vi "Rename Selected Waveform.vi"(8 "error in (no error)":errorcluster, 9 "New Waveform Name":string, 10 "Waveform Listbox Ref":refnum<vi>, 11 "Data In":T1 {"Toggle Channels"."Initial State" items=["High"=101, "Low"=102]; "Sample Rate" format="%.2p"}) -> (0 "error out":errorcluster, 3 "Data Out":T1 {"Toggle Channels"."Initial State" items=["High"=101, "Low"=102]; "Sample Rate" format="%.2p"})   [LabVIEW 2021]
uses:
  Controls/Data.ctl
  Controls/Script Trigger Routing.ctl
  Controls/Toggle Channel.ctl
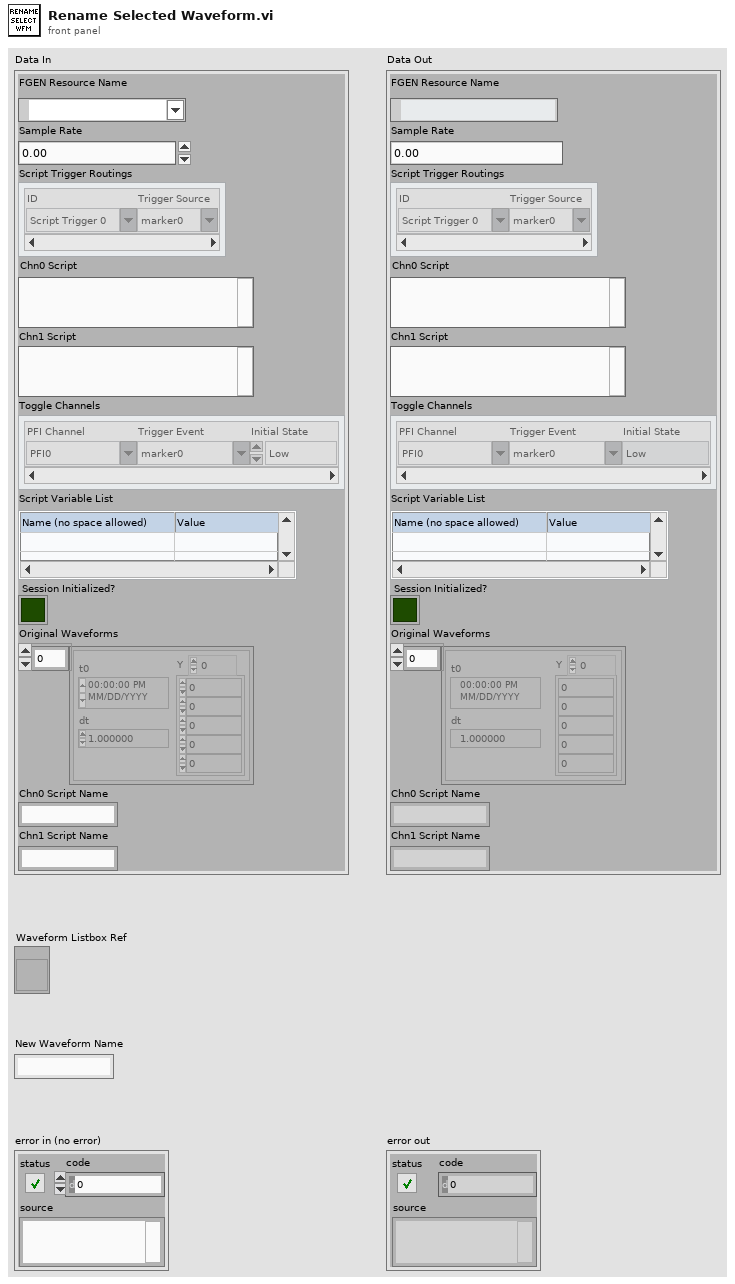
[diagram p1: front panel]
types:
  T1 = typedef "Data.ctl" = cluster{"FGEN Resource Name":refnum<k15>, "Sample Rate":dbl, "Script Trigger Routings":T2[], "Chn0 Script":string, "Chn1 Script":string, "Toggle Channels":T3[], "Script Variable List":string[][], "Session Initialized?":bool, "Original Waveforms":waveform(dbl)[], "Chn0 Script Name":string, "Chn1 Script Name":string}
  T2 = typedef "Script Trigger Routing.ctl" = cluster{"ID":string, "Trigger Source":string}
  T3 = typedef "Toggle Channel.ctl" = cluster{"PFI Channel":string, "Trigger Event":string, "Initial State":u16}
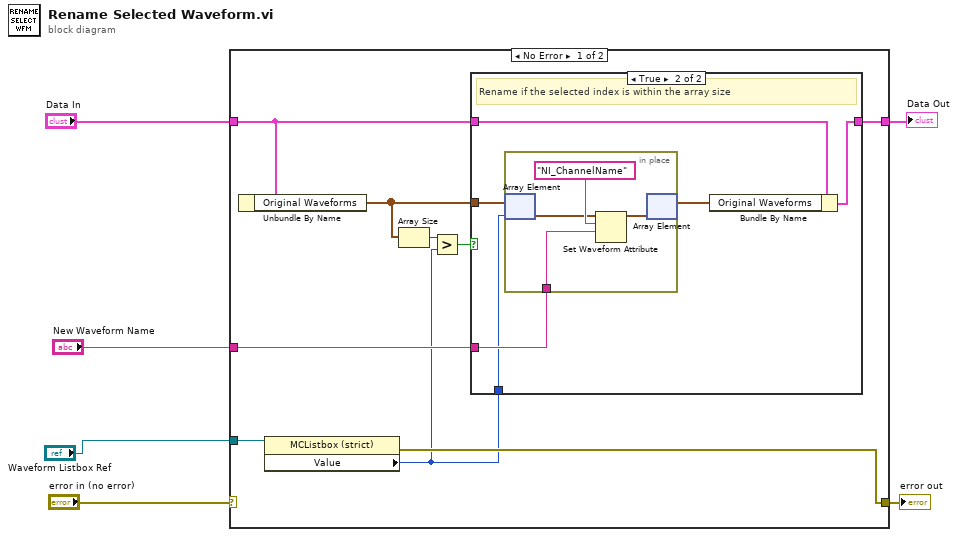
[diagram p0: block diagram]
diagram:
  n1 = case shown="No Error" "error in (no error)" {
    selector: "error in (no error)" -> [_ w28]
    tunnel: "Data In" -> [w15 w27]
    tunnel: [w11 w27] -> w5
    tunnel: [w13 w28] -> w3
    tunnel: "Waveform Listbox Ref" -> [w14 _]
    tunnel: "New Waveform Name" -> [w12 _]
    frame No Error {
      n2 = Unbundle By Name(w15) -> ("Original Waveforms"=w10:waveform(dbl)[])
      n3 = property class="MCListbox (strict)"(reference=w14) -> (error out=w13:errorcluster, "Value"=w8:i32)  [unwired: 1 in, 1 out]
      n4 = Array Size(array=w10) -> (size(s)=w9:i32)
      n5 = Greater?(x=w9, y=w8) -> (0:w7:bool)
      n6 = case shown="True" w7 {
        tunnel: w15 -> [w16 w22]
        tunnel: w12 -> [_ w21]
        tunnel: w8 -> [_ w20]
        tunnel: [w16 w17] -> w11
        tunnel: w10 -> [_ w18]
        frame False {
        }
        frame True {
          # "Rename if the selected index is within the array size"
          n7 = in-place {
            in-place-border: w21 -> [w25]
            n8 = in-place-array #1(w18, w20) -> (w24:waveform(dbl))
            n9 = Set Waveform Attribute(5:w25, 6:"NI_ChannelName", 7:w24) -> (3:w23:waveform(dbl))  [unwired: 1 in, 2 out]
            n10 = in-place-array #1(w23) -> (w19:waveform(dbl)[])  [unwired: 1 out]
          }
          n11 = Bundle By Name(cluster=w22, "Original Waveforms"=w19) -> (w17:T1)
        }
      }
    }
    frame Error {
    }
  }
  "Data Out" <- w5
  "error out" <- w3
